vi "Get Parent ID.vi"(7 "Linked List ID":string, 8 "error in (no error)":errorcluster, 11 "Linked List in":refnum<class "Linked List.lvclass">) -> (0 "error out":errorcluster, 1 "Valid Parent ID":bool, 2 "Parent ID":string, 3 "Linked List out":refnum<class "Linked List.lvclass">)   [LabVIEW 2020, in "Linked Lists.lvlib" / "Linked List.lvclass"]
uses:
  <vilib>/gpm_packages/@cs/linked-list/Source/Linked List/Linked List/Linked List.lvclass
  <vilib>/gpm_packages/@cs/linked-list/Source/Linked List/Linked List Definition/Linked List Definition.lvclass
  <vilib>/gpm_packages/@cs/linked-list/Source/Linked List/Linked List/Linked List.lvclass/Linked List.ctl
  <vilib>/gpm_packages/@cs/lookup-table/Source/LookupTable/LookupTable.lvclass/LookupTable.ctl
  3d7f4a9a-e650-4d06-8acf-6c8a7b50f671.vi
  <vilib>/gpm_packages/@cs/lookup-table/Source/LookupTable/Read Table Reference.vi
  3d7f4a9a-e650-4d06-8acf-6c8a7b50f671.vi/bdb305ec-b0a8-4a9c-bfcf-8ab8b20c2d64.vi
  <vilib>/gpm_packages/@cs/lookup-table/Source/LookupTable/LookupTable.lvclass
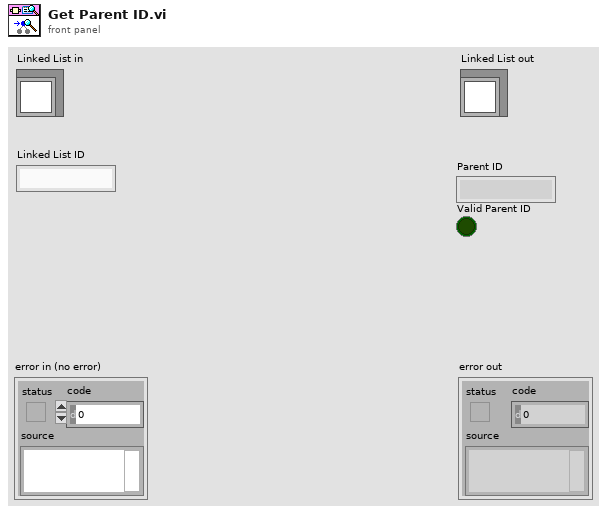
[diagram p1: front panel]
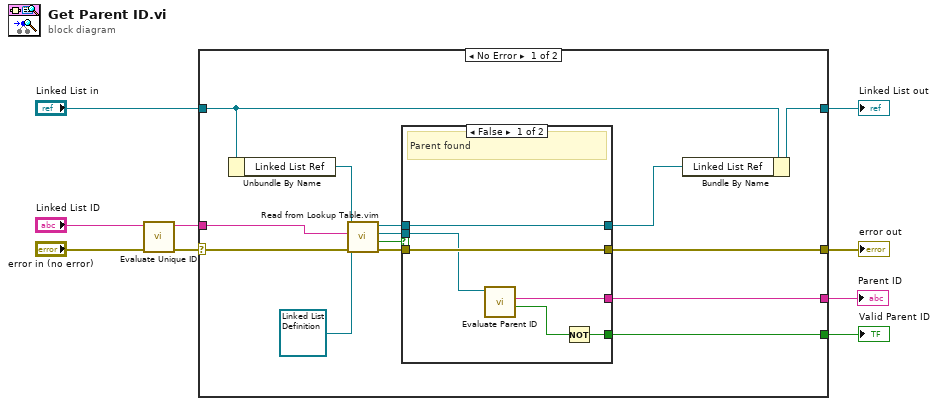
[diagram p0: block diagram]
diagram:
  n1 = call <vilib>:"Evaluate Unique ID.vi"("error in (no error)"="error in (no error)", "Unique ID"="Linked List ID") -> ("error out"=w7:errorcluster, "Unique ID Out"=w6:string)  [unwired: 8 in]
  n2 = case shown="No Error" w7 {
    selector: w7 -> [w23 w33]
    tunnel: w6 -> [w21 _]
    tunnel: "Linked List in" -> [w16 w32]
    tunnel: [w15 w32] -> w4
    tunnel: [w13 w33] -> w3
    tunnel: [w11 _] -> w2
    tunnel: [w10 _] -> w1
    frame No Error {
      n3 = Unbundle By Name(w16) -> ("Linked List Ref"=w22:refnum<data-value>)
      n4 = call "Read from Lookup Table.vim"("error in (no error)"=w23, "Type"=refnum<class "Linked List Definition.lvclass"> refnum ("Linked List.lvlib:Linked List Definition.lvclass"), "Item Name"=w21, "LookupTable Reference"=w22) -> ("error out"=w20:errorcluster, "Not Found?"=w12:bool, "Value"=w17:refnum<class "Linked List Definition.lvclass">, "LookupTable Reference Out"=w19:refnum<data-value>)  [unwired: 4 in]
      n5 = case shown="False" w12 {
        tunnel: w20 -> [w28 w30]
        tunnel: w19 -> [w29 w31]
        tunnel: w17 -> [w27 _]
        tunnel: [w29 w31] -> w14
        tunnel: [w28 w30] -> w13
        tunnel: [w26 _] -> w11
        tunnel: [w24 _] -> w10
        frame False {
          # "Parent found"
          n6 = call <vilib>:"Evaluate Parent ID.vi"("Linked List Definition in"=w27) -> ("Invalid Parent ID"=w25:bool, "Parent ID"=w26:string)  [unwired: 8 in, 1 out]
          n7 = Not(x=w25) -> (.not. x?=w24:bool)
        }
        frame True {
          # "Parent not found"
        }
      }
      n8 = Bundle By Name(cluster=w16, "Linked List Ref"=w14) -> (w15:refnum<class "Linked List.lvclass">)
    }
    frame Error {
    }
  }
  "error out" <- w3
  "Linked List out" <- w4
  "Parent ID" <- w2
  "Valid Parent ID" <- w1
